vi "Tosca-Apply Timeout to Output State.vi"(0 "State":refnum<class "State.lvclass">, 5 "AODO":T2, 9 "end on rep":bool, 11 "Trxn":i32, 12 "Trial type":T1) -> (4 "State out":refnum<class "State.lvclass">, 6 "AODO (out)":T2)   [LabVIEW 2020]
uses:
  Typedefs/Tosca-State AODO.ctl
  epl-vi-lib/Signal Synthesis VIs/4th Generation/Classes/SignalManager/SignalManager.lvclass
  Typedefs/Tosca-AO Runtime.ctl
  Typedefs/Tosca-DO Runtime.ctl
  Typedefs/Tosca-Event Type.ctl
  Classes/State/State.lvclass
  Classes/Timeout/Timeout.lvclass/Timeout.ctl
  Classes/Timeout/Read Units.vi
  Classes/Timeout/Read Expr.vi
  Classes/Timeout/Read Link to.vi
  Classes/Timeout/Timeout.lvclass
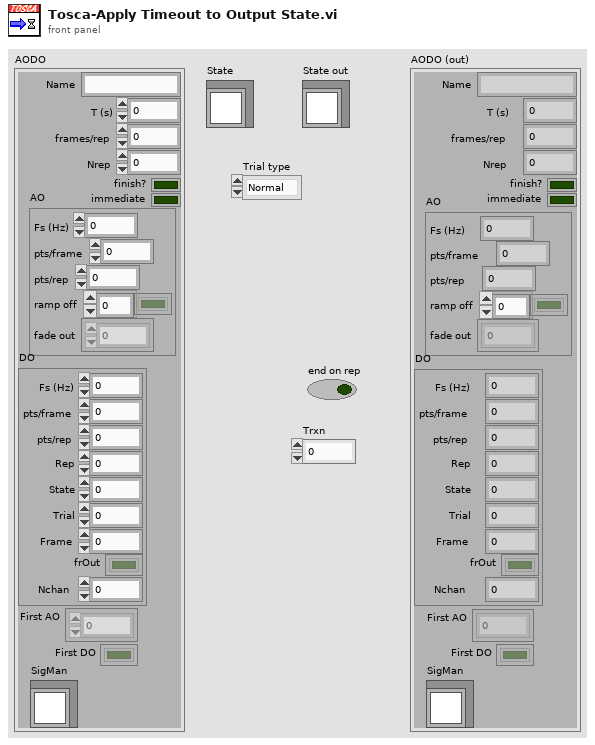
[diagram p1: front panel]
types:
  T1 = typedef "Tosca-Event Type.ctl" = enum16{"Normal", "CS+", "CS-"}
  T2 = typedef "Tosca-State AODO.ctl" = cluster{"Name":string, "T (s)":dbl, "First AO":dbl[][], "frames/rep":i32, "finish?":bool, "Nrep":i32, "AO":T3, "DO":T4, "immediate":bool, "First DO":bool[][], "SigMan":refnum<class "SignalManager.lvclass">}
  T3 = typedef "Tosca-AO Runtime.ctl" = cluster{"Fs (Hz)":dbl, "pts/frame":i32, "pts/rep":i32, "ramp off":bool[], "fade out":dbl[][]}
  T4 = typedef "Tosca-DO Runtime.ctl" = cluster{"Fs (Hz)":dbl, "pts/frame":i32, "pts/rep":i32, "Rep":i32, "State":i32, "Trial":i32, "Frame":i32, "frOut":bool[], "Nchan":i32}
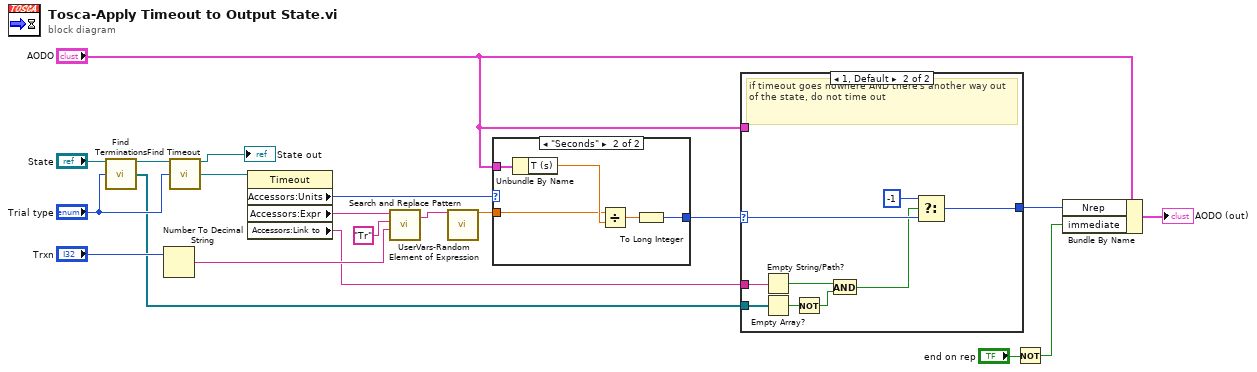
[diagram p0: block diagram]
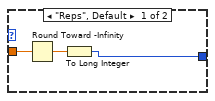
[diagram p2: hidden frame]
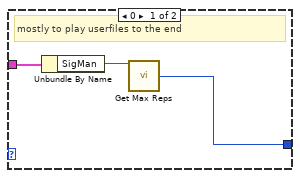
[diagram p3: hidden frame]
diagram:
  n1 = call "Find Terminations.vi"("State in"="State", "Type"="Trial type") -> ("State thru"=w4:refnum<class "State.lvclass">, "Terminations"=w1:refnum<class "Termination.lvclass">[])  [unwired: 11 in, 1 out]
  n2 = Number To Decimal String(number="Trxn") -> (decimal integer string=w12:string)  [unwired: 1 in]
  n3 = call "Find Timeout.vi"("State in"=w4, "Type"="Trial type") -> ("State thru"=→"State out":refnum<class "State.lvclass">, "Timeout"=w9:refnum<class "Timeout.lvclass">)  [unwired: 11 in, 1 out]
  n4 = property class="Timeout"(reference=w9) -> ("Accessors:Units"=w11:enum16{"Reps", "Seconds"}, "Accessors:Expr"=w10:string, "Accessors:Link to"=w6:string)  [unwired: 1 in, 2 out]
  n5 = call <vilib>:"Search and Replace Pattern.vi"("string"=w10, "regular expression (\"\")"="Tr" ("regular expression (\"\")"), "replace string (\"\")"=w12) -> ("result string"=w15:string)  [unwired: 2 in, 1 out]
  n6 = call "UserVars-Random Element of Expression.vi"("Expr"=w15) -> ("Random Element"=w17:dbl)  [unwired: 12 in, 2 out]
  n7 = case shown="\"Seconds\"" w11 {
    tunnel: [w21 w25] -> w16
    tunnel: "AODO" -> [_ w28]
    tunnel: w17 -> [w23 w24]
    frame "Reps", Default {
      n8 = Round Toward -Infinity(1:w23) -> (0:w22:dbl)
      n9 = To Long Integer(number=w22) -> (32bit integer=w21:i32)
    }
    frame "Seconds" {
      n10 = Unbundle By Name(w28) -> ("T (s)"=w27:dbl)
      n11 = Divide(x=w24, y=w27) -> (x/y=w26:dbl)
      n12 = To Long Integer(number=w26) -> (32bit integer=w25:i32)
    }
  }
  n13 = case shown="1, Default" w16 {
    selector: w16 -> [_ w39]
    tunnel: [w29 w33] -> w7
    tunnel: "AODO" -> [w31 _]
    tunnel: w6 -> [_ w40]
    tunnel: w1 -> [_ w37]
    frame 0 {
      # "mostly to play userfiles to the end"
      n14 = Unbundle By Name(w31) -> ("SigMan"=w30:refnum<class "SignalManager.lvclass">)
      n15 = call "Get Max Reps.vi"("SigMan in"=w30) -> ("max reps"=w29:i32)  [unwired: 12 in, 2 out]
    }
    frame 1, Default {
      # "if timeout goes nowhere AND there's another way out of the state, do not time out"
      n16 = Empty String/Path?(string/path=w40) -> (empty?=w36:bool)
      n17 = Empty Array?(array=w37) -> (empty?=w35:bool)
      n18 = Not(x=w35) -> (.not. x?=w34:bool)
      n19 = And(x=w36, y=w34) -> (x .and. y?=w32:bool)
      n20 = Select(t=-1, s=w32, f=w39) -> (s? t:f=w33:i32)
    }
  }
  n21 = Not(x="end on rep") -> (.not. x?=w18:bool)
  n22 = Bundle By Name(cluster="AODO", "Nrep"=w7, "immediate"=w18) -> (→"AODO (out)":T2)
